vi "write_dbl.vi"() -> ()   [LabVIEW 2019]
uses:
  <vilib>/RTI DDS Toolkit/Types/RTI DDS Advanced Writer Configuration.ctl
  <vilib>/RTI DDS Toolkit/VIs/AdvancedCreateWriter_NumDbl.vi
  <vilib>/RTI DDS Toolkit/VIs/Write_Num.vi
  <vilib>/RTI DDS Toolkit/Library/LVDDS_library.lvlib
panel:
  in  "Advanced Writer Configuration":T1={"typeName"="std_msgs::msg::dds_::Float32_", "keyName"="", "domainParticipantQoSProfile"="", "dataWriterQoSProfile"="", "forceArrayMapping?"=FALSE, "forceUnboundedString?"=FALSE}
  out "Waveform Chart":dbl(graph)=0.9214866621533888
  in  "Dial":u32(knob)=41 scale=0.0..100.0
  in  "stop":bool
  in  "Topic Name":string="rt/rosdbl"
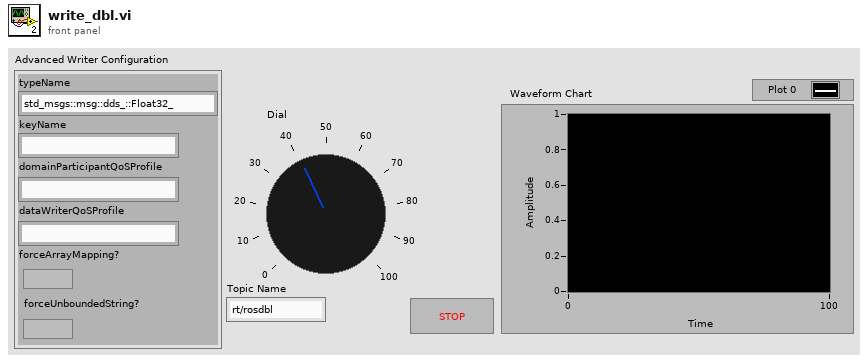
[diagram p1: front panel]
types:
  T1 = typedef "LVDDS_library.lvlib/RTI DDS Advanced Writer Configuration.ctl" = cluster{"typeName":string, "keyName":string, "domainParticipantQoSProfile":string, "dataWriterQoSProfile":string, "forceArrayMapping?":bool, "forceUnboundedString?":bool}
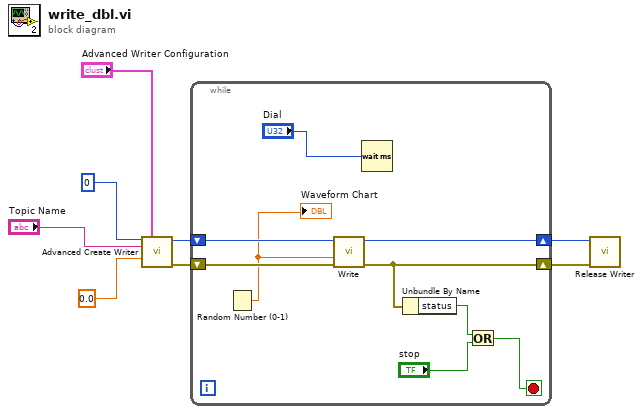
[diagram p0: block diagram]
diagram:
  n1 = call-poly <vilib>:"Advanced Create Writer.vi"("Domain Id"=u32 0, "Advanced Writer Configuration"="Advanced Writer Configuration", "Topic Name"="Topic Name", "Data Type"=0.0) -> ("DDS Object Ref"=w5:u64, "error out"=w8:errorcluster)  [unwired: 10 in]
  n2 = while {
    shift-right: [w14] -> w7
    shift-left: w8 -> [w17]
    shift-right: [w16] -> w6
    shift-left: w5 -> [w15]
    stop <- w11 stop-if-true
    n3 = Random Number (0-1)() -> (number: 0 to 1=w9:dbl)
    "Waveform Chart" <- w9
    n4 = call-poly <vilib>:"Write.vi"("error in (no error)"=w17, "Data"=w9, "DDS Object Ref in"=w15) -> ("error out"=w14:errorcluster, "DDS Object Ref out"=w16:u64)  [unwired: 7 in]
    n5 = Wait (ms)(milliseconds to wait="Dial") -> ()  [unwired: 1 out]
    n6 = Unbundle By Name(w14) -> ("status"=w12:bool)
    n7 = Or(x=w12, y="stop") -> (x .or. y?=w11:bool)
  }
  n8 = call <vilib>:"Release Writer.vi"("error in (no error)"=w7, "DDS Object Ref"=w6) -> ()  [unwired: 9 in, 1 out]
